vi "Colorbar1002.vi"   [LabVIEW 2013]
uses:
  <vilib>/Heliosphere Research LLC/Advanced Plotting Toolkit/Advanced Plotting Toolkit.lvlib
types:
  T1 = typedef "Advanced Plotting Toolkit.lvlib/PlotID.ctl" = i32
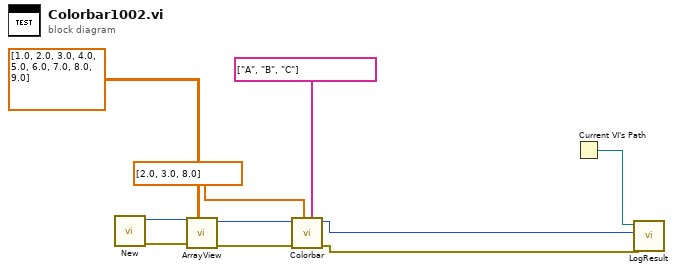
[diagram p0: block diagram]
diagram:
  n1 = call <vilib>:"New.vi"() -> ("error out"=w9:errorcluster, "Plot ID"=w8:T1)  [unwired: 10 in]
  n2 = call <vilib>:"ArrayView.vi"("Data"=dbl[][] [[1.0, 2.0, 3.0], [4.0, 5.0, 6.0], [7.0, 8.0, 9.0]], "error in (no error)"=w9, "Plot ID"=w8) -> ("error out"=w5:errorcluster, "Plot ID Out"=w6:T1)  [unwired: 7 in]
  n3 = call <vilib>:"Colorbar.vi"("Tick Labels"=string[] ["A", "B", "C"], "Ticks"=dbl[] [2.0, 3.0, 8.0], "error in (no error)"=w5, "Plot ID"=w6) -> ("error out"=w4:errorcluster, "Plot ID Out"=w3:T1)  [unwired: 6 in]
  n4 = Current VI's Path() -> (path=w10:path)
  n5 = call "LogResult.vi"("Test Result"=w4, "Test Artifact"=w3, "VI Path"=w10) -> ()  [unwired: 9 in]
